vi "32-bit to string.vi"() -> ()   [LabVIEW 2020]
panel:
  out "String":string
  out "Numeric":dbl
  out "binary":u32=1023 format="%.0b"
  in  "decimal 2":u32=1023 format="%.0b"
  in  "decimal":u32=1023 format="%.0b"
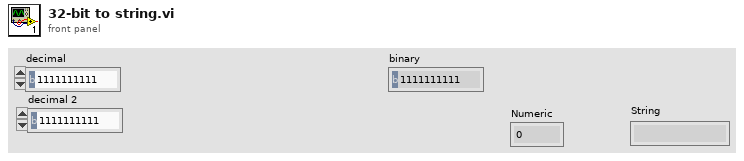
[diagram p1: front panel]
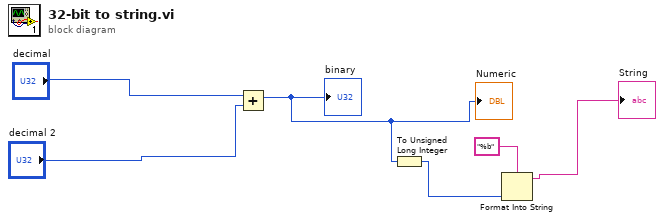
[diagram p0: block diagram]
diagram:
  n1 = Add(x="decimal", y="decimal 2") -> (x+y=w3:u32)
  "binary" <- w3
  "Numeric" <- w3
  n2 = To Unsigned Long Integer(number=w3) -> (unsigned 32bit integer=w4:u32)
  n3 = Format Into String(format string="%b", w4) -> (resulting string=→"String":string)  [unwired: 2 in, 1 out]
